vi "AddDateTimeMeasure.vi"(6 "MeasureExecutionStatus (NOT_COMPLETED)":T1=enum."NOT_COMPLETED", 7 "MeasureTime (Now)":timestamp, 8 "error in":errorcluster, 10 "Value":timestamp, 11 "StepRun in":refnum<class "StepRun.lvclass">) -> (0 "error out":errorcluster, 2 "RealMeasure":refnum<class "DateTimeMeasure.lvclass">, 3 "StepRun out":refnum<class "StepRun.lvclass">)   [LabVIEW 2021, in "ProligentXMLGenerator.lvlib" / "StepRun.lvclass"]
doc: "Add a Measure.\n\nDefines the value acquired by the measure.\nMeasures are globaly unique by their MeasureId property."
uses:
  StepRun.lvclass
  StepRun.lvclass/StepRun.ctl
  Measure/DateTimeMeasure/DateTimeMeasure.lvclass
  C:/Projects/proligent-xml-generator-labview/src/ProligentXMLGenerator/Measure/Measure/Measure.lvclass
  C:/Projects/proligent-xml-generator-labview/src/ProligentXMLGenerator/Measure/DateTimeMeasure/DateTimeMeasure.lvclass
  Base/ExecutionStatus/Value.ctl
  Base/ExecutionStatus/ExecutionStatus.lvclass
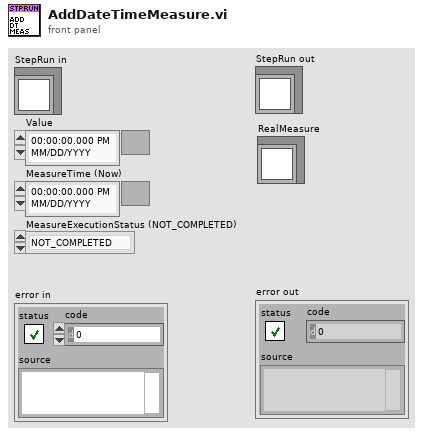
[diagram p1: front panel]
types:
  T1 = typedef "ProligentXMLGenerator.lvlib/ExecutionStatus.lvclass/Value.ctl" = enum16{"PASS", "FAIL", "NOT_COMPLETED", "ABORTED"}
  T2 = typedef "ProligentXMLGenerator.lvlib/StepRun.lvclass/Data.ctl" = cluster{"Name":string, "Measures":refnum<class "Measure.lvclass">[], "FailureReferences":refnum<class "FailureReference.lvclass">[], "Characteristics":refnum<class "Characteristic.lvclass">[], "Documents":refnum<class "Document.lvclass">[], "CustomData":refnum<class "CustomData.lvclass">, "StepExecutionStatus":refnum<class "ExecutionStatus.lvclass">, "StepRunId":refnum<class "Guid.lvclass">, "StepName":refnum<class "NonEmptyString_255.lvclass">, "StartDate":refnum<class "DateTime.lvclass">, "EndDate":refnum<class "DateTime.lvclass">, "TimeZoneInfoId":string}
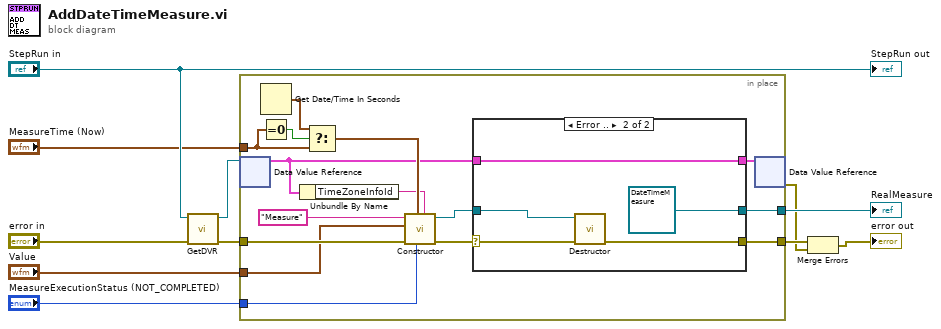
[diagram p0: block diagram]
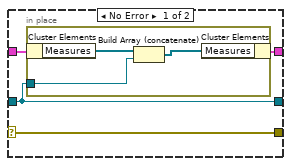
[diagram p2: hidden frame]
diagram:
  n1 = call "GetDVR.vi"("error in"="error in", "StepRun"="StepRun in") -> ("error out"=w5:errorcluster, "DVRReference"=w4:refnum<data-value>)  [unwired: 8 in]
  n2 = in-place "In Place Element Structure" {
    in-place-border: "Value" -> [w19]
    in-place-border: [w26] -> w6
    in-place-border: w5 -> [w20]
    in-place-border: [w24] -> w7
    in-place-border: "MeasureExecutionStatus (NOT_COMPLETED)" -> [w18]
    in-place-border: "MeasureTime (Now)" -> [w17]
    n3 = in-place-dvr #1(w4) -> (w13:T2)  [unwired: 1 out]
    n4 = Get Date/Time In Seconds() -> (seconds since 1Jan1904=w15:timestamp)
    n5 = Equal To 0?(x=w17) -> (x = 0?=w16:bool)
    n6 = Unbundle By Name(w13) -> ("TimeZoneInfoId"=w12:string)
    n7 = Select(t=w15, s=w16, f=w17) -> (s? t:f=w14:timestamp)
    n8 = call "Constructor.vi"("TimeZoneInfoId"=w12, "MeasureExecutionStatus"=w18, "MeasureTime"=w14, "error in"=w20, "Value"=w19, "Name"="Measure") -> ("error out"=w22:errorcluster, "DateTimeMeasure"=w23:refnum<class "DateTimeMeasure.lvclass">)  [unwired: 4 in]
    n9 = case shown="Error .." w22 {
      selector: w22 -> [w30 w37]
      tunnel: [w27 w38] -> w25
      tunnel: [w30 w36] -> w26
      tunnel: w23 -> [w29 w35]
      tunnel: w13 -> [w28 w38]
      tunnel: [w29 refnum<class "DateTimeMeasure.lvclass"> refnum ("ProligentResultProcessor:DateTimeMeasure")] -> w24
      frame No Error {
        n10 = in-place "In Place Element Structure" {
          in-place-border: w29 -> [w33]
          n11 = in-place-cluster #2(w28) -> ("Measures"=w32:refnum<class "Measure.lvclass">[])
          n12 = Build Array (concatenate)(w32, w33) -> (w31:refnum<class "Measure.lvclass">[])
          n13 = in-place-cluster #2("Measures"=w31) -> (w27:T2)
        }
      }
      frame Error {
        n14 = call "Destructor.vi"("error in"=w37, "DateTimeMeasure"=w35) -> ("error out"=w36:errorcluster)  [unwired: 9 in]
      }
    }
    n15 = in-place-dvr #1(w25) -> (w3:errorcluster)  [unwired: 1 out]
  }
  "RealMeasure" <- w7
  n16 = Merge Errors(w6, w3) -> (→"error out":errorcluster)
  "StepRun out" <- "StepRun in"
